vi "fpPrintScreen.vi"(7 "path to save image":path caption="image file path (leave empty to auto save in ~/Document/LabVIEW Data/data)", 8 "error in (no error)":errorcluster, 10 "flash sreen? (T)":bool=TRUE, 11 "VI ref":refnum<vi>) -> (0 "error out":errorcluster, 3 "image saved path":path)   [LabVIEW 2016]
doc: "Run the VI to screen print the Front Panel of the target VI into *.png file by wiring the target VI's <b>VI ref</b> as input. Assign a path to save the image from the input <b>image file path</b> or leave empty to save to ~/Document/LabVIEW Data/data. The file name is automatically generate in the following format like \"screen_print_2017_09_01_17_12_06.png\". Set <b>flash screen?</b> to FALSE to disable the screen flashing while screen printing of each this VI run."
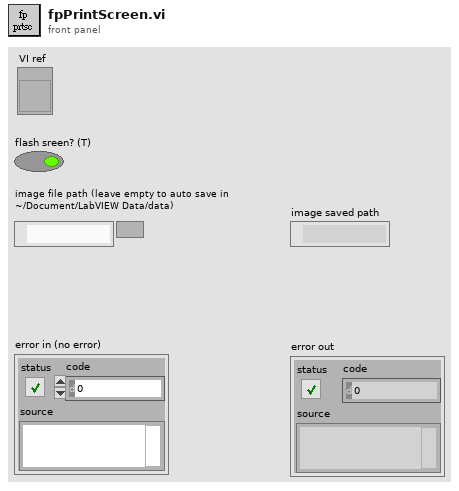
[diagram p1: front panel]
types:
  T1 = typedef "imagedata.ctl" = cluster{"image type":i32, "image depth":i32, "image":u8[], "mask":u8[], "colors":u32[], "Rectangle":cluster{"left":i16, "top":i16, "right":i16, "bottom":i16}}
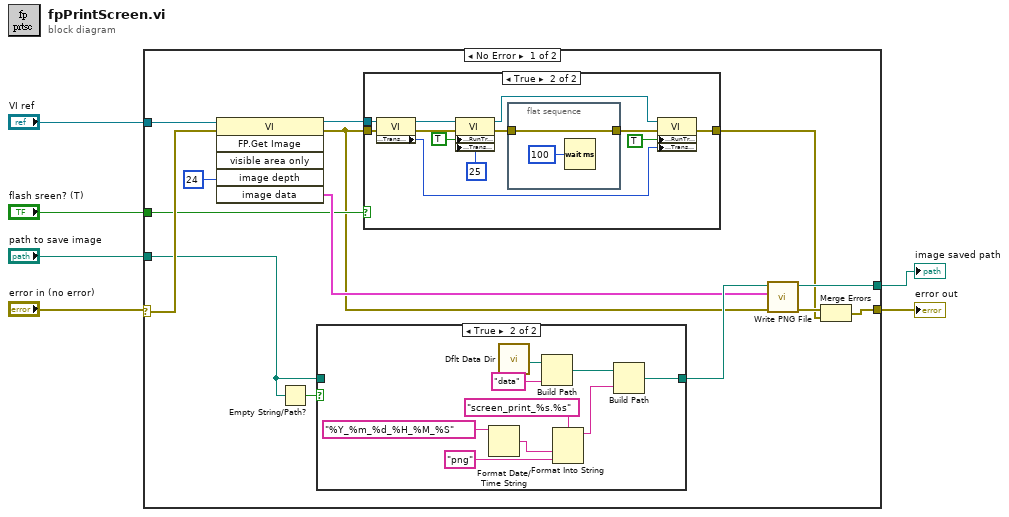
[diagram p0: block diagram]
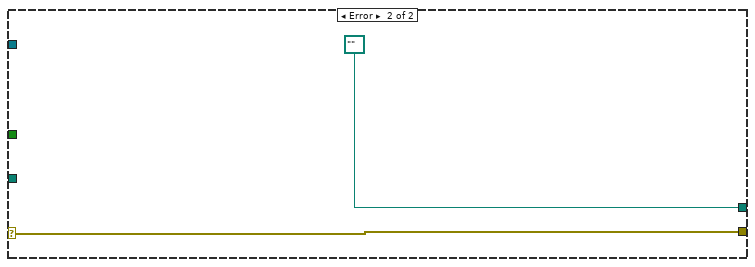
[diagram p4: hidden frame]
diagram:
  n1 = case shown="No Error" "error in (no error)" {
    selector: "error in (no error)" -> [w18 w47]
    tunnel: "VI ref" -> [w19 _]
    tunnel: [w8 w47] -> w4
    tunnel: [w14 path "" ("path")] -> w3
    tunnel: "flash sreen? (T)" -> [w12 _]
    tunnel: "path to save image" -> [w10 _]
    frame No Error {
      n2 = invoke class="VI" method="FP.Get Image"(reference=w19, error in=w18, "image depth"=24 ("Image Depth")) -> (reference out=w13:refnum<vi>, error out=w9:errorcluster, "image data"=w16:T1)  [unwired: 3 in, 3 out]
      n3 = Empty String/Path?(string/path=w10) -> (empty?=w11:bool)
      n4 = case shown="True" w11 {
        tunnel: [w21 w23] -> w17
        tunnel: w10 -> [w21 _]
        frame False {
        }
        frame True {
          n5 = Format Date/Time String(time format string (%c)="%Y_%m_%d_%H_%M_%S") -> (date/time string=w28:string)  [unwired: 2 in]
          n6 = call <vilib>:"Dflt Data Dir.vi"() -> ("App:Default Data Directory"=w26:path)
          n7 = Build Path(base path=w26, name or relative path="data") -> (appended path=w22:path)
          n8 = Format Into String(format string="screen_print_%s.%s", w28, "png" ("input 2")) -> (resulting string=w27:string)  [unwired: 2 in, 1 out]
          n9 = Build Path(base path=w22, name or relative path=w27) -> (appended path=w23:path)
        }
      }
      n10 = case shown="True" w12 {
        tunnel: w9 -> [w31 w37]
        tunnel: w13 -> [_ w36]
        tunnel: [w31 w34] -> w7
        frame False {
        }
        frame True {
          n11 = property class="VI"(reference=w36, error in=w37) -> (reference out=w43:refnum<vi>, error out=w42:errorcluster, "FP:Transparency"=w33:u8)
          n12 = property class="VI"(reference=w43, error in=w42, "FP:RunTransparently"=TRUE ("Front Panel Window:Run VI Transparently"), "FP:Transparency"=u8 25 ("Front Panel Window:Transparency")) -> (reference out=w35:refnum<vi>, error out=w41:errorcluster)
          n13 = flat-sequence {
            tunnel: [w45] -> w40
            tunnel: w41 -> [w45]
            frame #0 {
              n14 = Wait (ms)(milliseconds to wait=u32 100) -> ()  [unwired: 1 out]
            }
          }
          n15 = property class="VI"(reference=w35, error in=w40, "FP:RunTransparently"=TRUE ("Front Panel Window:Run VI Transparently"), "FP:Transparency"=w33) -> (error out=w34:errorcluster)  [unwired: 1 out]
        }
      }
      n16 = call <vilib>:"Write PNG File.vi"("error in (no error)"=w9, "image data"=w16, "path to PNG file"=w17) -> ("error out"=w15:errorcluster, "path"=w14:path)  [unwired: 7 in]
      n17 = Merge Errors(w15, w7) -> (w8:errorcluster)
    }
    frame Error {
    }
  }
  "error out" <- w4
  "image saved path" <- w3
